vi "Starter Kit 2.0 Roaming.vi"() -> ()   [LabVIEW 2018]
doc: "This VI demonstrates how to control the Robotics Starter Kit 2.0 robot. It is deployed to an sbRIO-9632, then run on the Real-Time controller."
uses:
  <vilib>/Studica/Studica Toolkit/Background/Mxp Selection.ctl
  <vilib>/robotics/Steering/Wheel/Rotation Direction.ctl
  <vilib>/robotics/Steering/Wheel/NI_Robotics_Wheel.lvclass
  <vilib>/robotics/Steering/Wheel/Wheel Parameters.ctl
  <vilib>/robotics/Steering/Steering Frame/NI_Robotics_Steering Frame.lvclass
  <vilib>/robotics/Utilities/Scan Angles/NI_Robotics_Scan Angles.lvlib
  <vilib>/robotics/Steering/Omnidirectional Wheel/Create Omnidirectional Wheel.vi
  <vilib>/robotics/Steering/Omnidirectional Wheel/NI_Robotics_Omnidirectional Wheel.lvclass
  <vilib>/robotics/Steering/Steering Frame/Create User Defined Steering Frame.vi
  <vilib>/Studica/Studica Toolkit/Background/PWM Channel.ctl
  <vilib>/Utility/AngleManip/NI_AngleManipulation.lvlib
  <vilib>/Utility/AngleManip/Degrees to Radians (Scalar SGL).vi
  <vilib>/Utility/AngleManip/Degrees to Radians (Scalar DBL).vi
  C:/Program Files (x86)/National Instruments/LabVIEW 2018/vi.lib/robotics/Steering/Wheel/NI_Robotics_Wheel.lvclass
panel:
  in  "milliseconds to wait":u32
  in  "stop":bool
  out "Sensor Data 2":cluster{"angles (deg)":dbl[], "distances":dbl[]}(graph)
  in  "Reset Encoders":bool
  out "Actual-SpeedList":dbl[](array[numeric])
  out "Tick Count(uSec) 2":u32=11529943 caption="Tick Count(Ticks)"
  in  "Motors":dbl[](array[numeric])
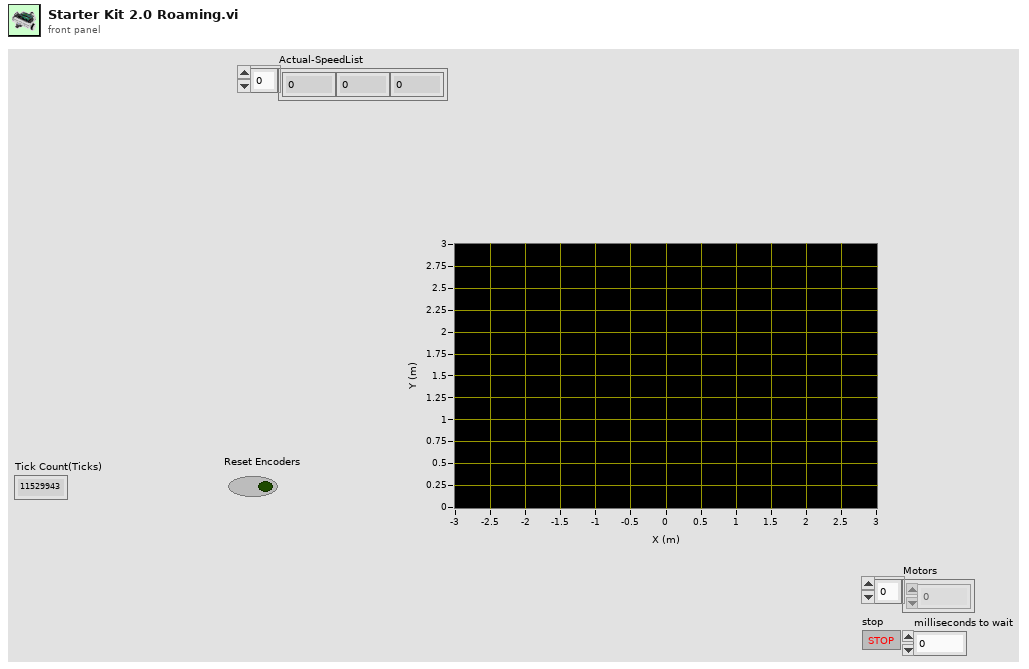
[diagram p1: front panel]
types:
  T1 = typedef "Mxp Selection.ctl" = enum16{"MXP A", "MXP B"}
  T2 = typedef "PWM Channel.ctl" = enum16{"Not Connected", "A/PWM0", "A/PWM1", "A/PWM2", "A/PWM3", "A/PWM4", "B/PWM0", "B/PWM1", "B/PWM2", "B/PWM3", "B/PWM4", "C/PWM0", "C/PWM1"}
  T3 = typedef "NI_Robotics_Wheel.lvclass/Wheel Parameters.ctl" = cluster{"wheel radius":dbl, "gear ratio":dbl, "forward rotation direction":T4}
  T4 = typedef "NI_Robotics_Wheel.lvclass/Rotation Direction.ctl" = u16
  T5 = typedef "NI_Robotics_Scan Angles.lvlib/Scan Angle Data.ctl" = cluster{"angles":dbl[], "distances":dbl[], "current index":i32, "previous index":i32}
  T6 = cluster{"PWM Channel":T2, "FPGA VI Reference Out":refnum<k20>}
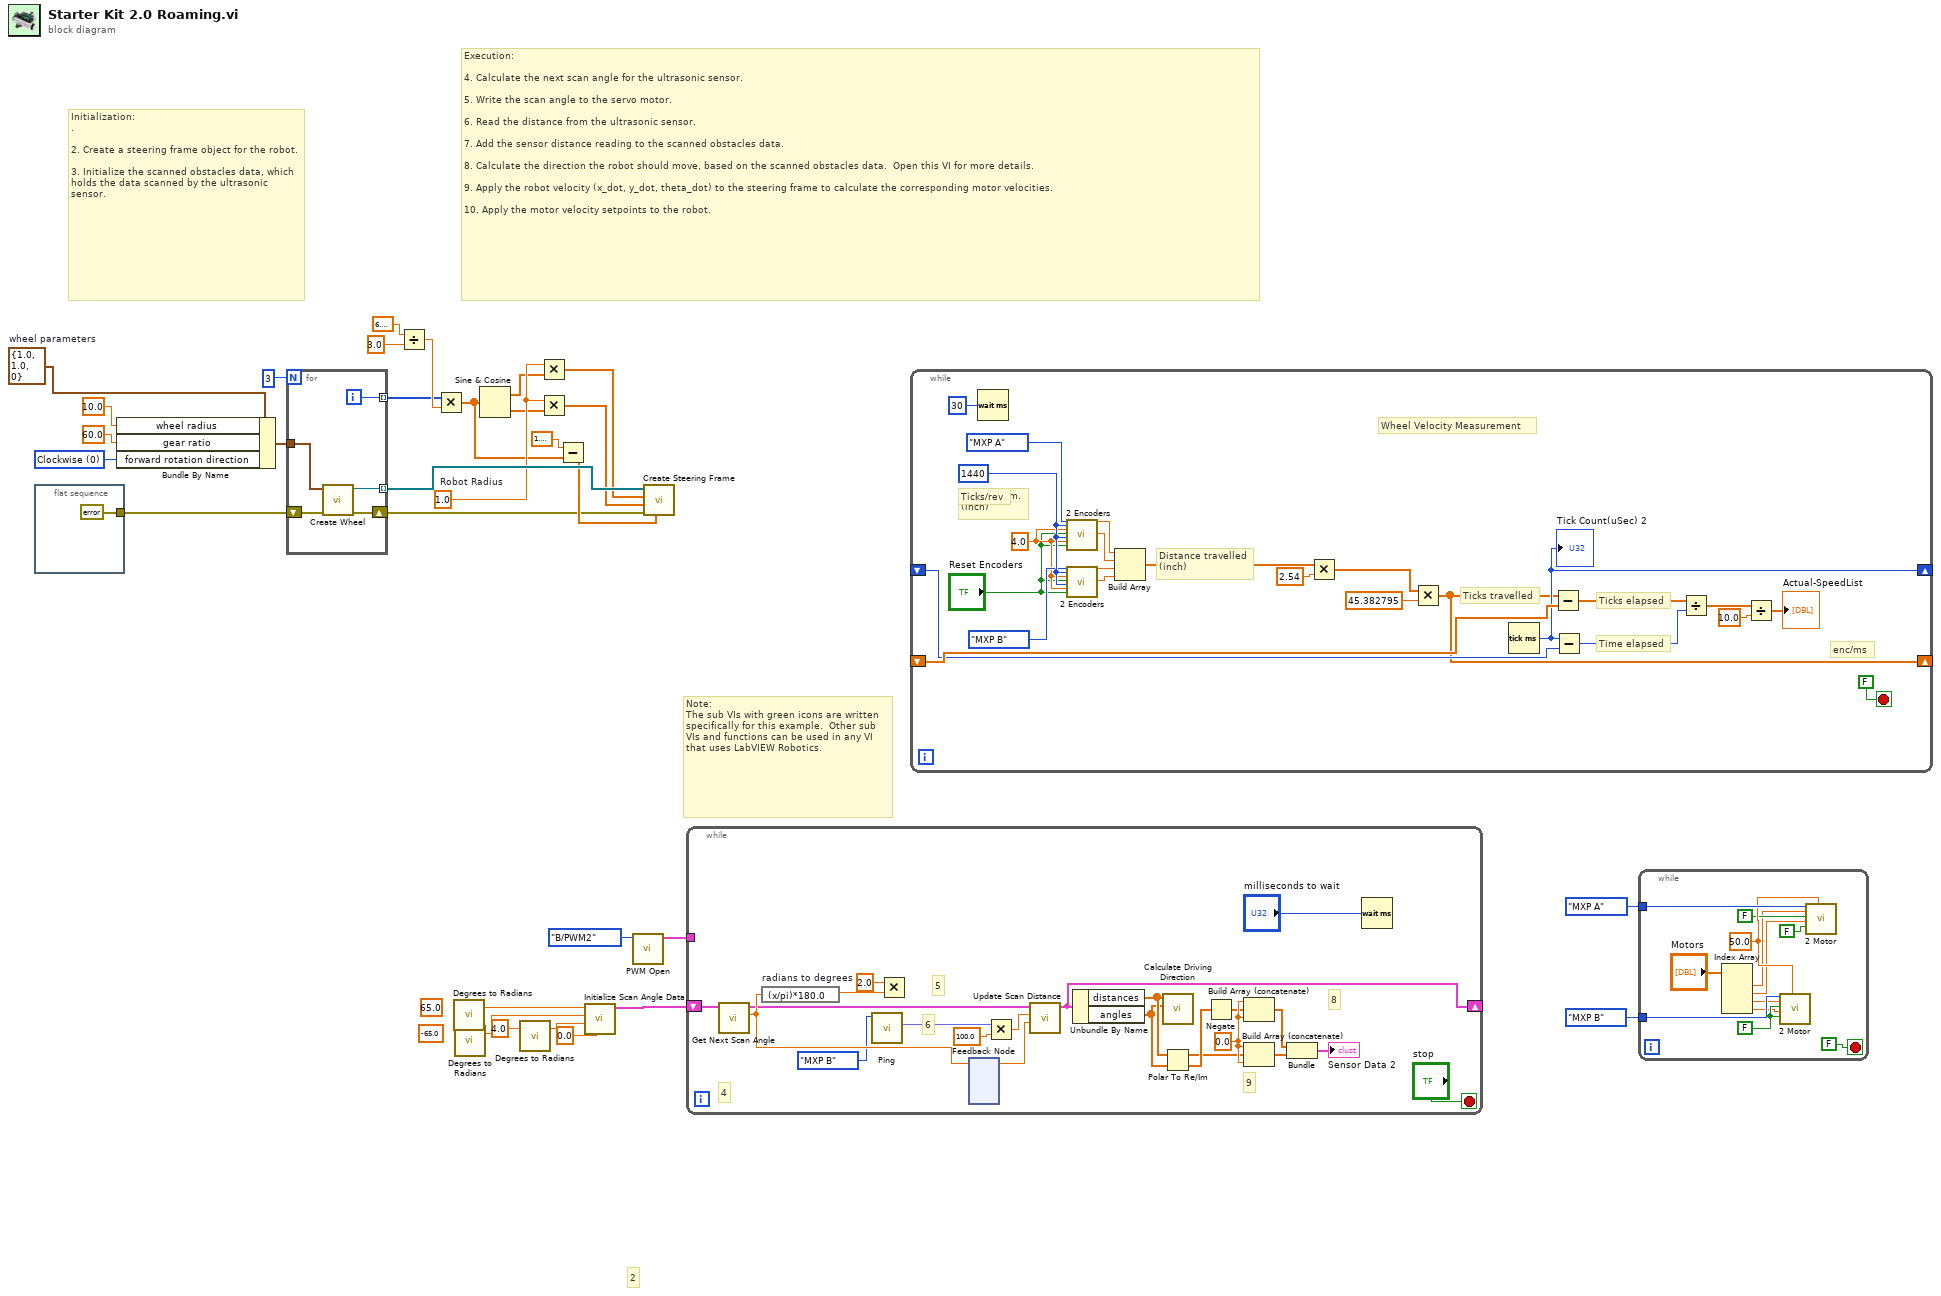
[diagram p0: block diagram]
diagram:
  (unwired) -65.0 ("min angle")
  (unwired) 65.0 ("max angle")
  w31 = T3 {"wheel radius"=1.0, "gear ratio"=1.0, "forward rotation direction"=0}  # wheel parameters
  w16 = T4 0 items=["Clockwise", "Counterclockwise"] ("forward rotation direction")
  w21 = 1.0  # Robot Radius
  # "Note:\nThe sub VIs with green icons are written specifically for this example.  Other sub VIs and functions can be used in any VI that uses LabVIEW Robotics."
  # "2"
  # "Execution:\n\n4. Calculate the next scan angle for the ultrasonic sensor.\n\n5. Write the scan angle to the servo motor.\n\n6. Read the distance from the ultrasonic sensor.\n\n7. Add the sensor distance reading to the scanned obstacles data.\n\n8. Calculate the direction the robot should move, based on the scanned obstacles data.  Open this VI for more details.\n\n9. Apply the robot velocity (x_dot, y_dot, theta_dot) to the steering frame to calculate the corresponding motor velocities.\n\n10. Apply the motor velocity setpoints to the robot."
  # "Initialization:\n.\n\n2. Create a steering frame object for the robot.\n\n3. Initialize the scanned obstacles data, which holds the data scanned by the ultrasonic sensor."
  n1 = flat-sequence {
    tunnel: [errorcluster {"status"=FALSE, "code"=0, "source"=""} ("error out")] -> w27
    frame #0 {
    }
  }
  n2 = Bundle By Name(cluster=w31, "wheel radius"=10.0, "gear ratio"=60.0, "forward rotation direction"=w16) -> (w28:T3)
  n3 = for {
    N: 3 -> [_]
    shift-right: [w36] -> w14
    shift-left: w27 -> [w37]
    tunnel: [w35] -> w26 mode=indexing
    tunnel: w28 -> [w34]
    tunnel: [w33] -> w22 mode=indexing
    i -> [w33]
    n4 = call-poly <vilib>:"Create Wheel.vi"("error in (no error)"=w37, "wheel parameters"=w34) -> ("error out"=w36:errorcluster, "omni wheel out"=w35:refnum<class "NI_Robotics_Omnidirectional Wheel.lvclass">)  [unwired: 8 in]
  }
  n5 = Divide(x=6.283185307179586, y=3.0) -> (x/y=w23:dbl)
  n6 = Multiply(x=w22, y=w23) -> (x*y=w11:dbl[])
  n7 = call-poly <vilib>:"Degrees to Radians.vi"() -> ("angle (rad)"=w10:sgl)  [unwired: 3 in]
  n8 = call-poly <vilib>:"Degrees to Radians.vi"() -> ("angle (rad)"=w7:sgl)  [unwired: 3 in]
  n9 = Sine & Cosine(0:w11) -> (1:w13:dbl[], 2:w12:dbl[])
  n10 = call-poly <vilib>:"Degrees to Radians.vi"("angle (deg)"=4.0 ("scan angle")) -> ("angle (rad)"=w8:dbl)  [unwired: 2 in]
  n11 = Multiply(x=w21, y=w13) -> (x*y=w20:dbl[])
  n12 = Multiply(x=w21, y=w12) -> (x*y=w19:dbl[])
  n13 = Subtract(x=1.5707963267948966, y=w11) -> (x-y=w17:dbl[])
  n14 = call <vilib>:"Initialize Scan Angle Data.vi"("initial angle (0)"=0.0, "scan angle"=w8, "min angle"=w7, "max angle"=w10) -> ("scan angles"=w4:T5)  [unwired: 6 in, 1 out]
  n15 = call <vilib>:"PWM Open.vi"("PWM Channel"=PWM_Channel."B/PWM2") -> ("PWM Info Out"=w3:T6)  [unwired: 9 in, 1 out]
  n16 = call-poly <vilib>:"Create Steering Frame.vi"("wheel frame angles (rad)"=w17, "error in (no error)"=w14, "wheel y positions"=w19, "wheel x positions"=w20, "wheels"=w26) -> ()  [unwired: 5 in, 2 out]
  n17 = while {
    shift-right: [w50] -> _
    shift-left: w4 -> [w53]
    tunnel: w3 -> [_]
    stop <- "stop" stop-if-true
    w48 = 0.0 ("element")
    # "9"
    # "8"
    # "6"
    # "5"
    # "4"
    n18 = call <vilib>:"Get Next Scan Angle.vi"("scan angles in"=w53) -> ("new angle"=w56:dbl, "scan angles out"=w52:T5)  [unwired: 9 in]
    n19 = expression code="(x/pi)*180.0" "radians to degrees"(w56) -> (w39:dbl)
    n20 = call <vilib>:"Ping.vi"("Mxp Side"=Mxp_Selection."MXP B") -> ("IN"=w54:fxp<+,64,16>)  [unwired: 8 in, 2 out]
    n21 = Multiply(x=2.0, y=w39) -> ()  [unwired: 1 out]
    n22 = feedback #1() -> (w59:dbl)  [unwired: 1 in]
    n23 = feedback-in #1(w56) -> ()
    n24 = Multiply(x=w54, y=100.0 ("default distance (NaN)")) -> (x*y=w57:dbl)
    n25 = call <vilib>:"Update Scan Distance.vi"("scan angle"=w59, "new scan distance"=w57, "scan angles in"=w52) -> ("scan angles out"=w50:T5)  [unwired: 8 in]
    n26 = Unbundle By Name(w50) -> ("distances"=w43:dbl[], "angles"=w42:dbl[])
    n27 = call "Calculate Driving Direction.vi"("obstacle angles (rad)"=w42, "obstacle distances (m)"=w43) -> ()  [unwired: 8 in, 2 out]
    n28 = Polar To Re/Im(2:w42, 3:w43) -> (0:w51:dbl[], 1:w44:dbl[])
    n29 = Negate(x=w51) -> (-x=w45:dbl[])
    n30 = Build Array (concatenate)(w48, w45, w48) -> (w49:dbl[])
    n31 = Build Array (concatenate)(w48, w44, w48) -> (w47:dbl[])
    n32 = Bundle(w49, w47) -> (→"Sensor Data 2":cluster{dbl[], dbl[]})  [unwired: 1 in]
    n33 = Wait (ms)(milliseconds to wait="milliseconds to wait") -> ()  [unwired: 1 out]
  }
  n34 = while {
    shift-right: [w66] -> _
    shift-left: _ -> [w71]
    shift-right: [w67] -> _
    shift-left: _ -> [w69]
    stop <- FALSE stop-if-true
    w64 = 4.0 ("Wheel Diameter M1 (inches)")
    w74 = u32 1440 ("Ticks Per Rev M0")
    # "Wheel Velocity Measurement"
    # "Ticks travelled"
    # "Distance travelled\n(inch)"
    # "Wheel diam.\n(inch)"
    # "Ticks/rev"
    # "Ticks elapsed"
    # "Time elapsed"
    # "enc/ms"
    n35 = Wait (ms)(milliseconds to wait=u32 30) -> ()  [unwired: 1 out]
    n36 = call <vilib>:"2 Encoders.vi"("Mxp Side"=Mxp_Selection."MXP A", "Ticks Per Rev M0"=w74, "Wheel Diameter M0 (inches)"=w64, "Reset Encoder 0"="Reset Encoders", "Ticks Per Rev M1"=w74, "Wheel Diameter M1 (inches)"=w64, "Reset Encoder 1"="Reset Encoders") -> ("Distance M0 (inches)"=w75:dbl, "Distance M1 (inches)"=w76:dbl)  [unwired: 18 in, 1 out]
    n37 = call <vilib>:"2 Encoders.vi"("Mxp Side"=Mxp_Selection."MXP B", "Ticks Per Rev M0"=w74, "Wheel Diameter M0 (inches)"=w64, "Reset Encoder 0"="Reset Encoders", "Ticks Per Rev M1"=w74, "Wheel Diameter M1 (inches)"=w64, "Reset Encoder 1"="Reset Encoders") -> ("Distance M0 (inches)"=w77:dbl, "Distance M1 (inches)"=w65:dbl)  [unwired: 18 in, 1 out]
    n38 = Build Array(w75, w76, w77, w65) -> (w79:dbl[])
    n39 = Multiply(x=w79, y=2.54) -> (x*y=w80:dbl[])
    n40 = Multiply(x=w80, y=45.382795) -> (x*y=w66:dbl[])
    n41 = Tick Count (ms)() -> (millisecond timer value=w67:u32)
    "Tick Count(uSec) 2" <- w67
    n42 = Subtract(x=w66, y=w71) -> (x-y=w70:dbl[])
    n43 = Subtract(x=w67, y=w69) -> (x-y=w82:u32)
    n44 = Divide(x=w70, y=w82) -> (x/y=w62:dbl[])
    n45 = Divide(x=w62, y=10.0) -> (x/y=→"Actual-SpeedList":dbl[])
  }
  n46 = while {
    tunnel: Mxp_Selection."MXP A" ("Mxp Side") -> [w95]
    tunnel: Mxp_Selection."MXP B" ("Mxp Side") -> [w94]
    stop <- FALSE stop-if-true
    w93 = 50.0 ("Frequency [Hz]")
    w89 = FALSE ("Invert M0")
    n47 = Index Array(array="Motors") -> (element #1=w87:dbl, element #2=w86:dbl, element #3=w85:dbl, element #4=w84:dbl)  [unwired: 4 in]
    n48 = call <vilib>:"2 Motor.vi"("Mxp Side"=w94, "Speed M0"=w85, "Invert M0"=w89, "Speed M1"=w84, "Invert M1"=w89, "Frequency [Hz]"=w93) -> ()  [unwired: 13 in, 1 out]
    n49 = call <vilib>:"2 Motor.vi"("Mxp Side"=w95, "Speed M0"=w87, "Invert M0"=FALSE, "Speed M1"=w86, "Invert M1"=FALSE ("Invert M0"), "Frequency [Hz]"=w93) -> ()  [unwired: 13 in, 1 out]
  }
